vi "Read Measurement (Adjacent Channel Power Ratio).vi"(0 "VISA resource name":refnum<visa-resource-name>, 5 "Maximum Time (120000 ms)":i32=120000, 11 "error in (no error)":errorcluster) -> (3 "Main Channel Power(dBm)":dbl, 4 "VISA resource name out":refnum<visa-resource-name>, 6 "Upper Adjacent Channel Power(dBm)":dbl[](array[numeric]), 8 "Low Adjacent Channel Power(dBm)":dbl[](array[numeric]), 10 "Upper Adjacent Channel Power Ratio(dB)":dbl[](array[numeric]), 14 "Low Adjacent Channel Power Ratio(dB)":dbl[](array[numeric]), 15 "error out":errorcluster)   [LabVIEW 2022 SP3, in "Agilent N934X Series.lvlib"]
doc: "Returns the results of last measurement(Adjacent Channel Power Ratio) and does not initiate data acquisition."
uses:
  <instrlib>/Agilent N934X Series/Agilent N934X Series.lvlib
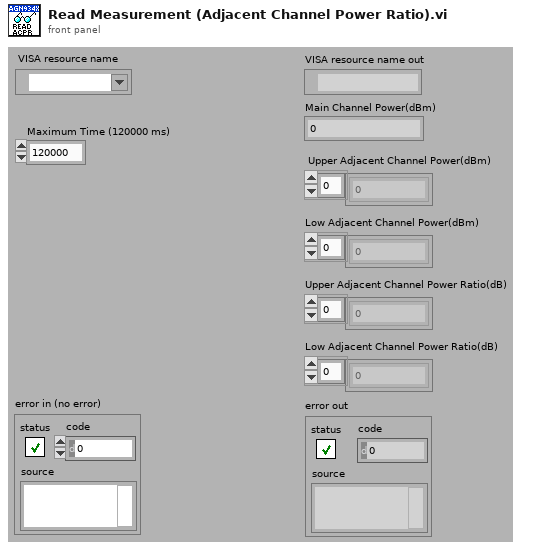
[diagram p1: front panel]
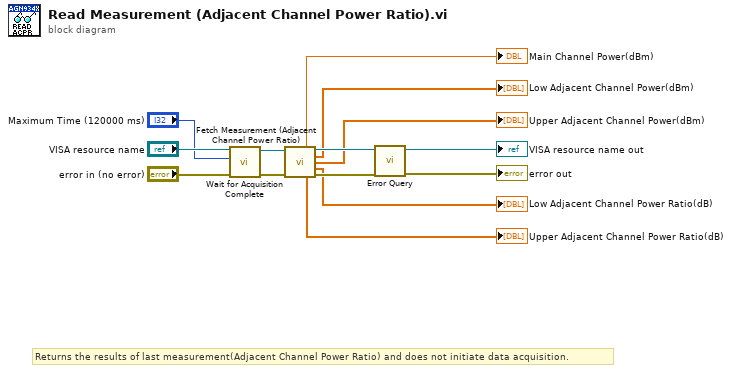
[diagram p0: block diagram]
diagram:
  # "Returns the results of last measurement(Adjacent Channel Power Ratio) and does not initiate data acquisition."
  n1 = call <instrlib>:"Wait for Acquisition Complete.vi"("error in (no error)"="error in (no error)", "Maximum Time (10000 ms)"="Maximum Time (120000 ms)", "VISA resource name"="VISA resource name") -> ("error out"=w9:errorcluster, "VISA resource name out"=w11:refnum<visa-resource-name>)  [unwired: 7 in]
  n2 = call <instrlib>:"Fetch Measurement (Adjacent Channel Power Ratio).vi"("VISA resource name"=w11, "error in (no error)"=w9) -> ("Main Channel Power(dBm)"=→"Main Channel Power(dBm)":dbl, "VISA resource name out"=w7:refnum<visa-resource-name>, "Low Adjacent Channel Power(dBm)"=→"Low Adjacent Channel Power(dBm)":dbl[], "Upper Adjacent Channel Power Ratio(dB)"=→"Upper Adjacent Channel Power(dBm)":dbl[], "Low Adjacent Channel Power Ratio(dB)"=→"Low Adjacent Channel Power Ratio(dB)":dbl[], "Upper Adjacent Channel Power(dBm)"=→"Upper Adjacent Channel Power Ratio(dB)":dbl[], "error out"=w6:errorcluster)  [unwired: 7 in]
  n3 = call <instrlib>:"Error Query.vi"("error in (no error)"=w6, "VISA resource name"=w7) -> ("error out"=→"error out":errorcluster, "VISA resource name out"=→"VISA resource name out":refnum<visa-resource-name>)  [unwired: 6 in, 2 out]
